vi "PSP-Nx-Remote.vi"(1 "Connection":T1=enum."1" caption="Port") -> (7 "X_Left":i32 caption="Left X" format="%#_3e", 13 "Y_Left":i32 caption="Left Y", 18 "X_Right":i32 caption="Right X" format="%.3e", 19 "Y_Right":i32 caption="Right Y" format="%.3p")   [LabVIEW 2009]
uses:
  mindsensors.com LVHS Toolkit/Resources/Library.llb/PadSelectorInput.ctl
  mindsensors.com LVHS Toolkit/Resources/Library.llb/MerlotRadioButton.ctl
panel:
  in  "Address":u8=2
  # "mindsensors.com\nCopyright (c) 2009 by mindsensors.com\nEmail: info (<at>) mindsensors (<dot>) com\n\nThis program is free software. You can redistribute it and/or modify\nit under the terms of the GNU General Public License as published by\nthe Free Software Foundation; version 3 of the License.\nRead the license at: http://www.gnu.org/licenses/gpl.txt"
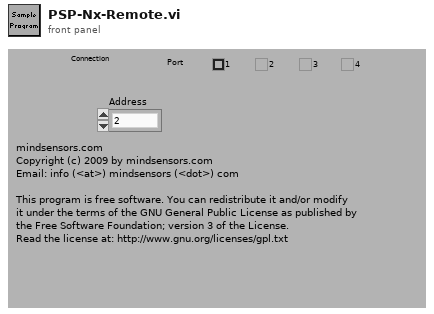
[diagram p1: front panel]
types:
  T1 = typedef "PadSelectorInput.ctl" = enum32{"0", "1", "2", "3", "4"}
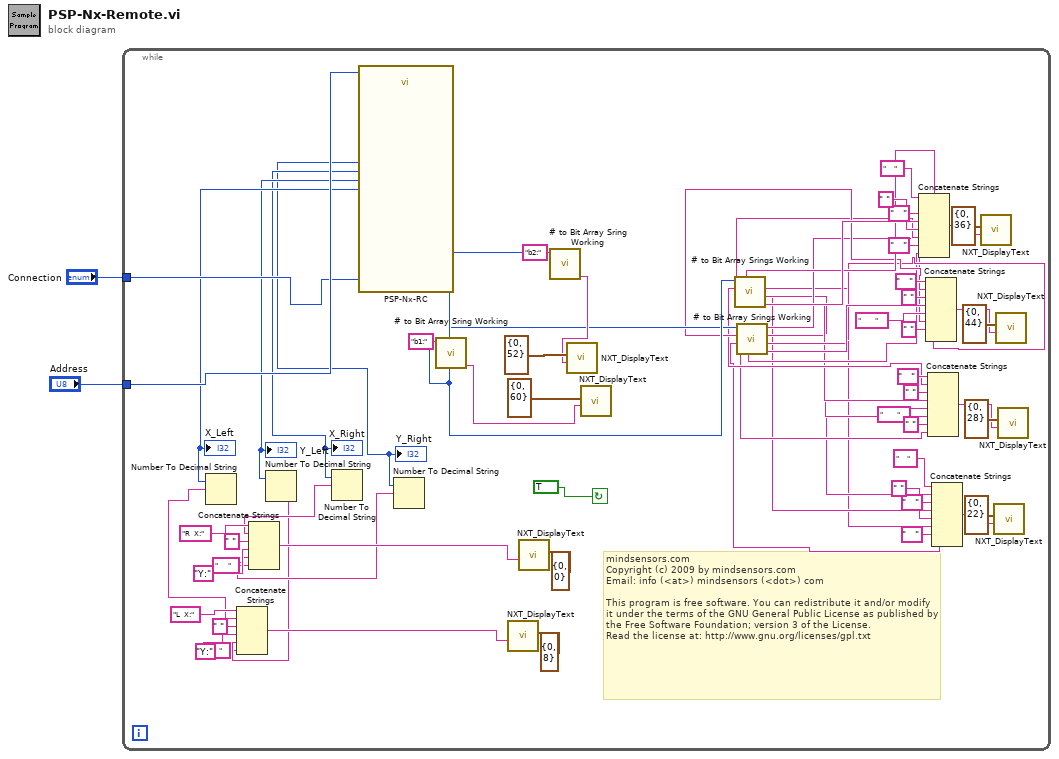
[diagram p0: block diagram]
diagram:
  n1 = while {
    tunnel: "Address" -> [w73]
    tunnel: "Connection" -> [w72]
    stop <- TRUE continue-if-true
    # "mindsensors.com\nCopyright (c) 2009 by mindsensors.com\nEmail: info (<at>) mindsensors (<dot>) com\n\nThis program is free software. You can redistribute it and/or modify\nit under the terms of the GNU General Public License as published by\nthe Free Software Foundation; version 3 of the License.\nRead the license at: http://www.gnu.org/licenses/gpl.txt"
    n2 = call "PSP-Nx-RC.vi"("Connection"=w72, "Address"=w73) -> ("last_left_X"=w6:i32, "last_left_Y"=w5:i32, "last_b_1"=w48:u8, "last_right_X"=w4:i32, "last_b_2"=w47:u8, "last_right_Y"=w3:i32)  [unwired: 2 in, 18 out]
    "X_Left" <- w6
    "Y_Left" <- w5
    "X_Right" <- w4
    "Y_Right" <- w3
    n3 = Number To Decimal String(number=w6) -> (decimal integer string=w61:string)  [unwired: 1 in]
    n4 = Number To Decimal String(number=w5) -> (decimal integer string=w54:string)  [unwired: 1 in]
    n5 = Concatenate Strings("L  X:" ("string"), w61, " " ("string"), "Y:" ("string"), w54, "     " ("string")) -> (w63:string)
    n6 = Number To Decimal String(number=w4) -> (decimal integer string=w65:string)  [unwired: 1 in]
    n7 = Number To Decimal String(number=w3) -> (decimal integer string=w57:string)  [unwired: 1 in]
    n8 = Concatenate Strings("R  X:" ("string"), w65, " " ("string"), "Y:" ("string"), w57, "     " ("string")) -> (w67:string)
    n9 = call "# to Bit Array Sring Working.vi"("Number"=w48, "Choose String"="b1:") -> ("Final String"=w49:string)  [unwired: 8 in]
    n10 = call "NXT_DisplayText.vi"("Text"=w63, "Location (0,0)"=cluster{"X":i16, "Y":i16} {"X"=0, "Y"=8}) -> ()  [unwired: 9 in, 1 out]
    n11 = call "NXT_DisplayText.vi"("Text"=w67, "Location (0,0)"=cluster{"X":i16, "Y":i16} {"X"=0, "Y"=0}) -> ()  [unwired: 9 in, 1 out]
    n12 = call "# to Bit Array Sring Working.vi"("Number"=w47, "Choose String"="b2:") -> ("Final String"=w52:string)  [unwired: 8 in]
    n13 = call "NXT_DisplayText.vi"("Text"=w52, "Location (0,0)"=cluster{"X":i16, "Y":i16} {"X"=0, "Y"=52}) -> ()  [unwired: 9 in, 1 out]
    n14 = call "NXT_DisplayText.vi"("Text"=w49, "Location (0,0)"=cluster{"X":i16, "Y":i16} {"X"=0, "Y"=60}) -> ()  [unwired: 9 in, 1 out]
    n15 = call "# to Bit Array Srings Working.vi"("Number"=w48) -> ("P1"=w14:string, "P1 2"=w10:string, "P1 3"=w13:string, "P1 4"=w20:string, "P1 5"=w16:string, "P1 6"=w8:string, "P1 7"=w9:string, "P1 8"=w22:string)  [unwired: 2 in]
    n16 = call "# to Bit Array Srings Working.vi"("Number"=w47) -> ("P1"=w12:string, "P1 2"=w7:string, "P1 3"=w11:string, "P1 4"=w17:string, "P1 5"=w15:string, "P1 6"=w19:string, "P1 7"=w18:string, "P1 8"=w21:string)  [unwired: 2 in]
    n17 = Concatenate Strings("    " ("string"), w20, "   " ("string"), w22, " " ("string"), w16, "   " ("string"), w17) -> (w28:string)
    n18 = Concatenate Strings("   " ("string"), w19, " " ("string"), w21, "       " ("string"), w15, " " ("string"), w18) -> (w33:string)
    n19 = Concatenate Strings("   " ("string"), w14, " " ("string"), w13, "       " ("string"), w12, " " ("string"), w11) -> (w45:string)
    n20 = Concatenate Strings("    " ("string"), w10, "   " ("string"), w9, " " ("string"), w8, "   " ("string"), w7) -> (w40:string)
    n21 = call "NXT_DisplayText.vi"("Text"=w28, "Location (0,0)"=cluster{"X":i16, "Y":i16} {"X"=0, "Y"=36}) -> ()  [unwired: 9 in, 1 out]
    n22 = call "NXT_DisplayText.vi"("Text"=w40, "Location (0,0)"=cluster{"X":i16, "Y":i16} {"X"=0, "Y"=22}) -> ()  [unwired: 9 in, 1 out]
    n23 = call "NXT_DisplayText.vi"("Text"=w33, "Location (0,0)"=cluster{"X":i16, "Y":i16} {"X"=0, "Y"=44}) -> ()  [unwired: 9 in, 1 out]
    n24 = call "NXT_DisplayText.vi"("Text"=w45, "Location (0,0)"=cluster{"X":i16, "Y":i16} {"X"=0, "Y"=28}) -> ()  [unwired: 9 in, 1 out]
  }
